vi "Score_Update.vi"(1 "Score":i16, 4 "Player":u8) -> ()   [LabVIEW 2018]
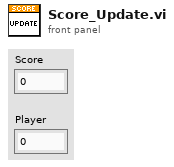
[diagram p1: front panel]
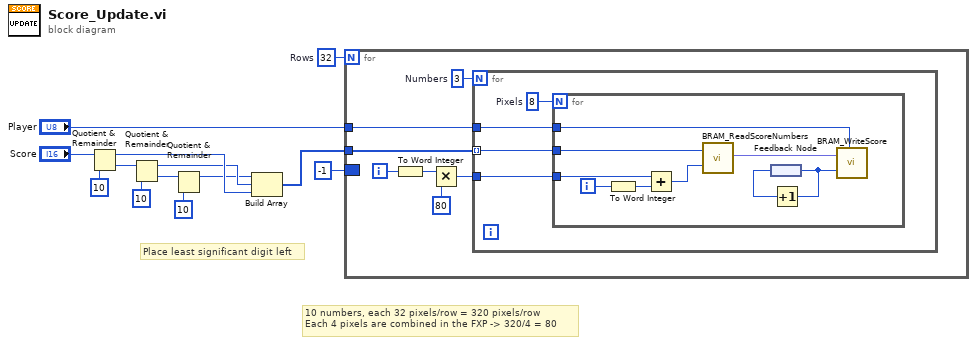
[diagram p0: block diagram]
diagram:
  w4 = 32  # Rows
  # "10 numbers, each 32 pixels/row = 320 pixels/row\nEach 4 pixels are combined in the FXP -> 320/4 = 80"
  # "Place least significant digit left"
  n1 = Quotient & Remainder(x="Score", y=i16 10) -> (x-y*floor(x/y)=w13:i16, floor(x/y)=w9:i16)
  n2 = Quotient & Remainder(x=w9, y=i16 10) -> (x-y*floor(x/y)=w5:i16, floor(x/y)=w7:i16)
  n3 = Quotient & Remainder(x=w7, y=i16 10) -> (x-y*floor(x/y)=w2:i16)  [unwired: 1 out]
  n4 = Build Array(w2, w5, w13) -> (w1:i16[])
  n5 = for {
    N: w4 -> [_]
    tunnel: "Player" -> [w20]
    tunnel: w1 -> [w17]
    border: i16 -1 -> [_]
    i -> [w19]
    w18 = 3  # Numbers
    n6 = To Word Integer(number=w19) -> (16bit integer=w16:i16)
    n7 = Multiply(x=w16, y=i16 80) -> (x*y=w14:i16)
    n8 = for {
      N: w18 -> [_]
      tunnel: w20 -> [w24]
      tunnel: w17 -> [w21] mode=indexing
      tunnel: w14 -> [w22]
      w23 = 8  # Pixels
      n9 = for {
        N: w23 -> [_]
        tunnel: w24 -> [w33]
        tunnel: w22 -> [w31]
        tunnel: w21 -> [w29]
        i -> [w32]
        n10 = To Word Integer(number=w32) -> (16bit integer=w30:i16)
        n11 = Add(x=w31, y=w30) -> (x+y=w28:i16)
        n12 = call "BRAM_ReadScoreNumbers.vi"("Number"=w29, "Address"=w28) -> ("PixelData"=w25:fxp<+,4,4>)  [unwired: 17 in]
        n13 = feedback #1() -> (w27:i16)
        n14 = Increment(x=w27) -> (x+1=w26:i16)
        n15 = feedback-in #1(w26) -> ()
        n16 = call "BRAM_WriteScore.vi"("Data"=w25, "Address"=w26, "Player"=w33) -> ()  [unwired: 17 in]
      }
    }
  }
